vi "set hot pixel correction.vi"(8 "error in (no error)":errorcluster, 11 "Thorcam in":refnum<class "Thorcam.lvclass">) -> (0 "error out":errorcluster, 3 "Thorcam out":refnum<class "Thorcam.lvclass">)   [LabVIEW 2012, in "Thorcam.lvclass"]
uses:
  Thorcam.lvclass
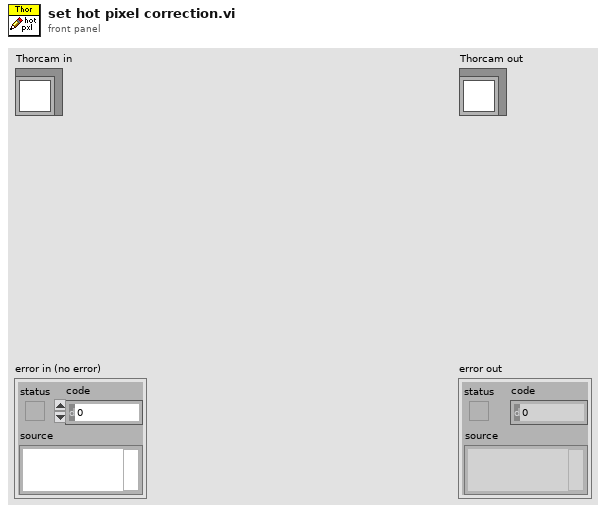
[diagram p1: front panel]
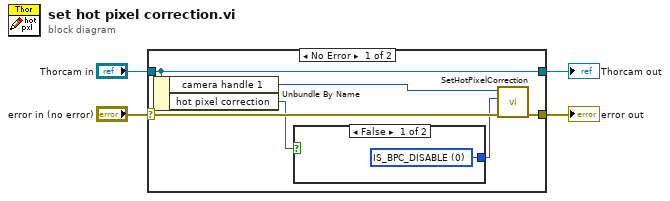
[diagram p0: block diagram]
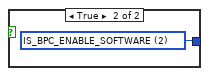
[diagram p2: hidden frame]
diagram:
  n1 = case shown="No Error" "error in (no error)" {
    selector: "error in (no error)" -> [w8 w14]
    tunnel: [w7 w14] -> w3
    tunnel: [w10 w13] -> w1
    tunnel: "Thorcam in" -> [w10 w13]
    frame No Error {
      n2 = Unbundle By Name(w10) -> ("camera handle 1"=w9:u32, "hot pixel correction"=w5:bool)
      n3 = case shown="False" w5 {
        tunnel: [w11 w12] -> w6
        frame False {
          w11 = 0 items=["IS_BPC_DISABLE"=0, "IS_BPC_ENABLE_SOFTWARE"=2, "IS_GET_BPC_MODE"=32768] ("Mode")
        }
        frame True {
          w12 = 2 items=["IS_BPC_DISABLE"=0, "IS_BPC_ENABLE_SOFTWARE"=2, "IS_GET_BPC_MODE"=32768] ("Mode")
        }
      }
      n4 = call <instrlib>:"SetHotPixelCorrection.vi"("error in"=w8, "Mode"=w6, "Camera Handle In"=w9) -> ("error out"=w7:errorcluster)  [unwired: 6 in, 2 out]
    }
    frame Error {
    }
  }
  "error out" <- w3
  "Thorcam out" <- w1
